vi "SH_Execl.vi"(0 "report in":refnum<class "NI_report.lvclass">, 1 "border? (F)":bool, 2 "font":T1={"font name"="", "font size"=10.0, "bold"=0, "italic"=0, "underline"=0, "strike through"=0, "font color"=16777216} {"font size" format="%0.2f"; "strike through" items=["Unchanged", "Yes", "No"]; "underline" items=["Unchanged", "Yes", "No"]; "italic" items=["Unchanged", "Yes", "No"]; "bold" items=["Unchanged", "Yes", "No"]}, 3 "font settings source":u16(ring) items=["VI Inputs", "Font Dialog Box"], 5 "text":string, 7 "start (-1, -1)":cluster{"row":i32, "column":i32}={"row"=-1, "column"=-1}, 9 "end (-1, -1)":cluster{"row":i32, "column":i32}={"row"=-1, "column"=-1}, 11 "error in (no error)":errorcluster, 12 "name (\"\")":string) -> (4 "report out":refnum<class "NI_report.lvclass">, 6 "font out":T1={"font name"="", "font size"=10.0, "bold"=0, "italic"=0, "underline"=0, "strike through"=0, "font color"=16777216} {"font size" format="%0.2f"; "strike through" items=["Unchanged", "Yes", "No"]; "underline" items=["Unchanged", "Yes", "No"]; "italic" items=["Unchanged", "Yes", "No"]; "bold" items=["Unchanged", "Yes", "No"]}, 8 "next cell bottom-left":cluster{"row":i32, "column":i32}, 10 "next cell top-right":cluster{"row":i32, "column":i32}, 15 "error out":errorcluster)   [LabVIEW 2015]
uses:
  <vilib>/Utility/NIReport.llb/NI_report.lvclass
  <vilib>/addons/_office/_exclsub.llb/font.ctl
  <vilib>/addons/_office/NI_ReportGenerationToolkit.lvlib
  <vilib>/Utility/NIReport.llb/Excel/NI_Excel.lvclass
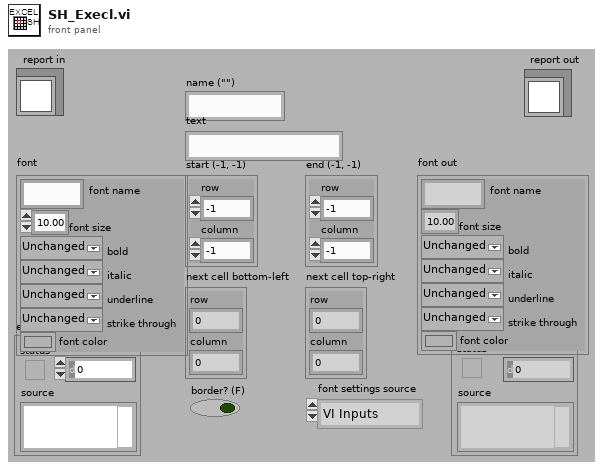
[diagram p1: front panel]
types:
  T1 = typedef "NI_ReportGenerationToolkit.lvlib/font.ctl" = cluster{"font name":string, "font size":dbl, "bold":u16, "italic":u16, "underline":u16, "strike through":u16, "font color":u32}
  T2 = cluster{"on/off":bool, "weight":i32, "color":u32}
  T3 = cluster{"Charset (-1)":i16, "Weight (-1)":i16, "Name":string, "Size":string}
  T4 = cluster{"position (Excel)":cluster{"row":i32, "column":i32}, "name (Excel)":string, "bookmark (Word)":string}
  T5 = cluster{"italic":u16, "strike through":u16, "underline":u16, "bold":u16}
  T6 = cluster{i32, i32, i32, i32, "charset":i16, "weight":i16, "name":string, "size":string, "text color":u32}
  T7 = typedef "NI_ReportGenerationCore.lvlib/font.ctl" = cluster{"font name":string, "font size":dbl, "bold":u16, "italic":u16, "underline":u16, "strike through":u16, "font color":u32}
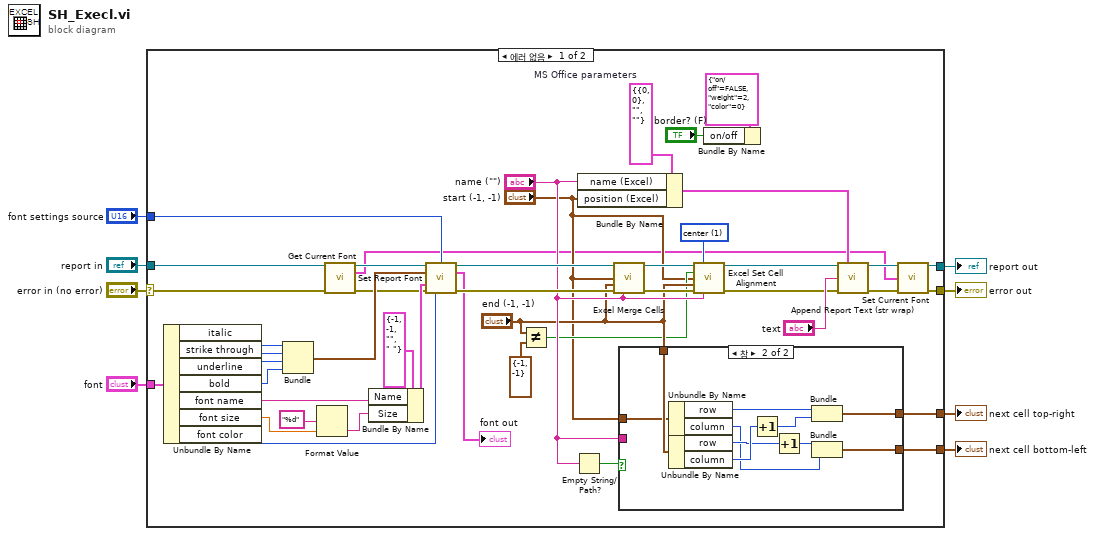
[diagram p0: block diagram]
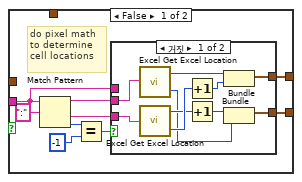
[diagram p2: hidden frame]
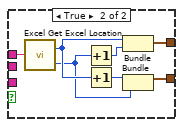
[diagram p3: hidden frame]
diagram:
  n1 = case shown="에러 없음" "error in (no error)" {
    selector: "error in (no error)" -> [w19 w89]
    tunnel: "font" -> [w35 _]
    tunnel: [w34 _] -> w7
    tunnel: [w33 _] -> w6
    tunnel: "report in" -> [w22 w90]
    tunnel: [w12 w89] -> w4
    tunnel: [w13 w90] -> w3
    tunnel: "font settings source" -> [w21 _]
    frame No Error {
      w50 = T4 {"position (Excel)"={"row"=0, "column"=0}, "name (Excel)"="", "bookmark (Word)"=""}  # MS Office parameters
      w30 = 1 items=["top", "center", "bottom"] ("vertical alignment")
      n2 = Unbundle By Name(w35) -> ("italic"=w40:u16, "strike through"=w43:u16, "underline"=w42:u16, "bold"=w41:u16, "font name"=w39:string, "font size"=w45:dbl, "font color"=w36:u32)
      n3 = Bundle("italic"=w40, "strike through"=w43, "underline"=w42, "bold"=w41) -> (w37:T5)  [unwired: 1 out]
      n4 = Format Value(format string="%d", value (0)=w45) -> (output string=w38:string)  [unwired: 1 out]
      n5 = call <vilib>:"Get Current Font.vi"("report in"=w22, "error in (no error)"=w19) -> ("report.lvclass"=w23:refnum<class "NI_report.lvclass">, "font"=w11:T6, "error out"=w24:errorcluster)  [unwired: 11 out]
      n6 = Bundle By Name(cluster=T3 {"Charset (-1)"=-1, "Weight (-1)"=-1, "Name"="", "Size"=" "} ("font settings"), "Name"=w39, "Size"=w38) -> (w52:T3)
      n7 = call-dynamic "Set Report Font.vi"("report in"=w23, "text color (unchanged)"=w36, "font settings source (VI Inputs)"=w21, "text options"=w37, "font settings"=w52, "error in (no error)"=w24) -> ("report out"=w49:refnum<class "NI_report.lvclass">, "font out"=→"font out":T7, "error out"=w48:errorcluster)  [unwired: 7 in]
      n8 = Not Equal?(x="end (-1, -1)", y=cluster{"row":i32, "column":i32} {"row"=-1, "column"=-1}) -> (x != y?=w25:bool)
      n9 = Empty String/Path?(string/path="name (\"\")") -> (empty?=w29:bool)
      n10 = Bundle By Name(cluster=w50, "name (Excel)"="name (\"\")", "position (Excel)"="start (-1, -1)") -> (w16:T4)
      n11 = call <vilib>:"Excel Merge Cells.vi"("report in"=w49, "start (-1, -1)"="start (-1, -1)", "end (-1, -1)"="end (-1, -1)", "error in (no error)"=w48, "name (\"\")"="name (\"\")") -> ("report out"=w31:refnum<class "NI_report.lvclass">, "error out"=w32:errorcluster)  [unwired: 9 out]
      n12 = case shown="참" w29 {
        tunnel: "end (-1, -1)" -> [_ w82]
        tunnel: [w56 w81] -> w34
        tunnel: [w55 w80] -> w33
        tunnel: "start (-1, -1)" -> [_ w79]
        tunnel: "name (\"\")" -> [w57 _]
        frame False {
          # "do pixel math\nto determine\ncell locations"
          n13 = Match Pattern(string=w57, regular expression=":") -> (before substring=w54:string, after substring=w53:string, offset past match=w60:i32)  [unwired: 2 out]
          n14 = Equal?(x=w60, y=-1) -> (x = y?=w58:bool)
          n15 = case shown="거짓" w58 {
            tunnel: w57 -> [_ w78]
            tunnel: [w66 w76] -> w56
            tunnel: [w62 w72] -> w55
            tunnel: w54 -> [w71 _]
            tunnel: w53 -> [w70 _]
            frame False {
              n16 = call <vilib>:"Excel Get Excel Location.vi"("cell's name"=w71) -> ("row"=w69:i32, "column"=w63:i32)
              n17 = call <vilib>:"Excel Get Excel Location.vi"("cell's name"=w70) -> ("row"=w65:i32, "column"=w68:i32)
              n18 = Increment(x=w68) -> (x+1=w67:i32)
              n19 = Increment(x=w65) -> (x+1=w64:i32)
              n20 = Bundle("row"=w69, w67) -> (w66:cluster{"row":i32, i32})  [unwired: 1 out]
              n21 = Bundle(w64, "column"=w63) -> (w62:cluster{i32, "column":i32})  [unwired: 1 out]
            }
            frame True {
              n22 = call <vilib>:"Excel Get Excel Location.vi"("cell's name"=w78) -> ("row"=w75:i32, "column"=w74:i32)
              n23 = Increment(x=w74) -> (x+1=w77:i32)
              n24 = Increment(x=w75) -> (x+1=w73:i32)
              n25 = Bundle("row"=w75, w77) -> (w76:cluster{"row":i32, i32})  [unwired: 1 out]
              n26 = Bundle(w73, "column"=w74) -> (w72:cluster{i32, "column":i32})  [unwired: 1 out]
            }
          }
        }
        frame True {
          n27 = Unbundle By Name(w79) -> ("row"=w88:i32, "column"=w83:i32)
          n28 = Unbundle By Name(w82) -> ("row"=w85:i32, "column"=w87:i32)
          n29 = Increment(x=w87) -> (x+1=w86:i32)
          n30 = Increment(x=w85) -> (x+1=w84:i32)
          n31 = Bundle("row"=w88, w86) -> (w81:cluster{"row":i32, i32})  [unwired: 1 out]
          n32 = Bundle(w84, "column"=w83) -> (w80:cluster{i32, "column":i32})  [unwired: 1 out]
        }
      }
      n33 = call <vilib>:"Excel Set Cell Alignment.vi"("report in"=w31, "vertical alignment (top)"=w30, "wrap text? (F)"=w25, "start (-1, -1)"="start (-1, -1)", "end (-1, -1)"="end (-1, -1)", "error in (no error)"=w32, "name (\"\")"="name (\"\")") -> ("report out"=w10:refnum<class "NI_report.lvclass">, "error out"=w9:errorcluster)  [unwired: 1 in, 6 out]
      n34 = Bundle By Name(cluster=T2 {"on/off"=FALSE, "weight"=2, "color"=0} ("inside border"), "on/off"="border? (F)") -> ()  [unwired: 1 out]
      n35 = call <vilib>:"Append Report Text (str wrap).vi"("report in"=w10, "MS Office parameters"=w16, "text"="text", "error in (no error)"=w9) -> ("report out"=w14:refnum<class "NI_report.lvclass">, "error out"=w15:errorcluster)  [unwired: 2 in, 8 out]
      n36 = call <vilib>:"Set Current Font.vi"("report in"=w14, "font"=w11, "error in (no error)"=w15) -> ("report out"=w13:refnum<class "NI_report.lvclass">, "error out"=w12:errorcluster)  [unwired: 11 out]
    }
    frame Error {
    }
  }
  "report out" <- w3
  "error out" <- w4
  "next cell bottom-left" <- w6
  "next cell top-right" <- w7
